vi "Read.vi"(8 "error in (no error)":errorcluster, 11 "Error Command Config in":refnum<class "Error Command Config.lvclass">) -> (0 "error out":errorcluster, 2 "Message":string, 3 "Error Command Config out":refnum<class "Error Command Config.lvclass">)   [LabVIEW 2020, in "VolatusSeqConfig.lvlib" / "Error Command Config.lvclass"]
uses:
  Error Command Config.lvclass
  Error Command Config.lvclass/Error Command Config.ctl
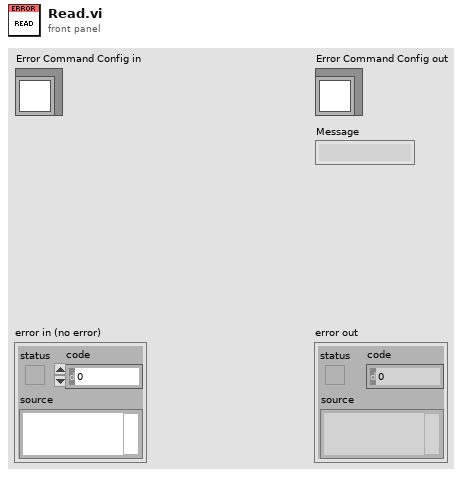
[diagram p1: front panel]
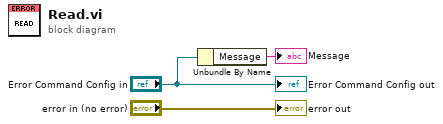
[diagram p0: block diagram]
diagram:
  n1 = Unbundle By Name("Error Command Config in") -> ("Message"=→"Message":string)
  "error out" <- "error in (no error)"
  "Error Command Config out" <- "Error Command Config in"
